vi "Handle Error.vi"(8 "error in (no error)":errorcluster, 11 "IMediator In":refnum<class "IMediator.lvclass">) -> (0 "error out":errorcluster, 2 "stop actor?":bool=TRUE, 3 "IMediator Out":refnum<class "IMediator.lvclass">)   [LabVIEW 2017, in "IMediator.lvlib" / "IMediator.lvclass"]
doc: "(<B>Filename</B>: Actor Framework.lvlib:Actor.lvclass:Handle Error.vi)\n\nDefines how the actor handles an error that occurred while processing a message. By default, this method does nothing except stop the actor."
uses:
  IMediator.lvclass
  gpm_packages/@cs/event-logger/Source/Composed Log/Log Sink/Log Level.ctl
  gpm_packages/@cs/event-logger/Source/Composed Log/Log Sink/Log Sink.lvclass
  gpm_packages/@cs/event-logger/Source/Composed Log/Composed Log.lvlib
  <vilib>/ActorFramework/Actor/Actor.lvclass
  C:/Program Files (x86)/National Instruments/LabVIEW 2017/vi.lib/ActorFramework/Actor/Actor.lvclass
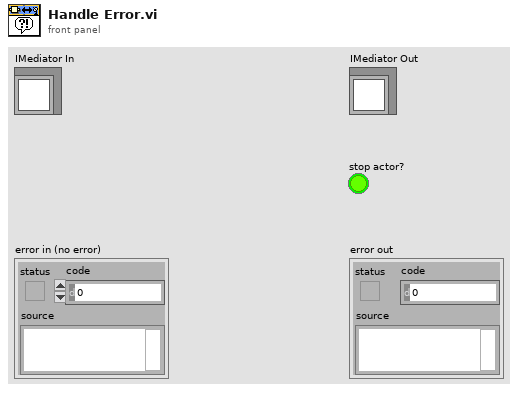
[diagram p1: front panel]
types:
  T1 = typedef "Composed Log.lvlib/Log Sink.lvclass/Log Level.ctl" = enum16{"Debug", "Info", "Warning", "Error", "Critical"}
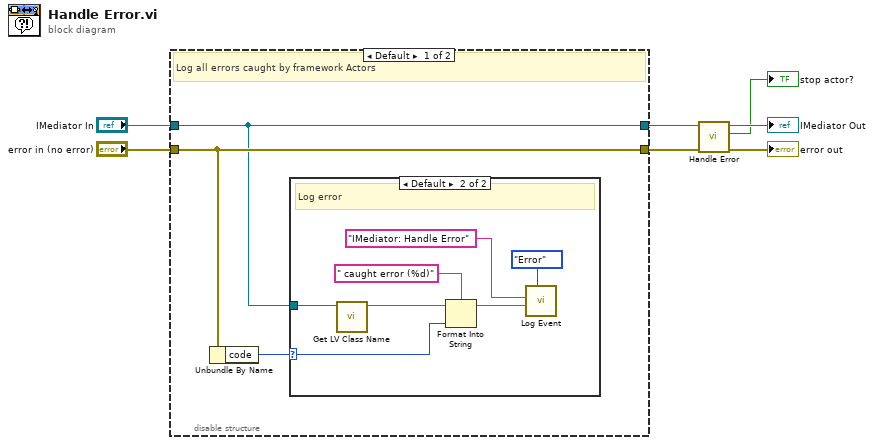
[diagram p0: block diagram]
diagram:
  n1 = disable-structure shown="Default" {
    disable-tunnel: "IMediator In" -> [w8 w19]
    disable-tunnel: [w8 w19] -> w2
    disable-tunnel: "error in (no error)" -> [w10 w18]
    disable-tunnel: [w10 w18] -> w1
    frame condition #0 (active) {
      # "Log all errors caught by framework Actors"
      n2 = Unbundle By Name(w10) -> ("code"=w9:i32)
      n3 = case shown="Default" w9 {
        selector: w9 -> [_ w14]
        tunnel: w8 -> [_ w13]
        frame 43 {
          # "Normal shutdown -- Do not log"
        }
        frame Default {
          # "Log error"
          n4 = call <vilib>:"Get LV Class Name.vi"("object"=w13) -> ("class name"=w16:string)  [unwired: 9 in, 1 out]
          n5 = Format Into String(format string=" caught error (%d)", initial string=w16, w14) -> (resulting string=w11:string)  [unwired: 1 in, 1 out]
          n6 = call "Log Event.vi"("Event Level"=Log_Level."Error", "Data To Log"=w11, "SourceID"="IMediator: Handle Error") -> ()  [unwired: 7 in, 2 out]
        }
      }
    }
    frame condition #1 {
      # "Remove all logging from this method at compile time"
    }
  }
  n7 = call-parent "Handle Error.vi"("error in (no error)"=w1, "Actor in"=w2) -> ("error out"=→"error out":errorcluster, "stop actor?"=→"stop actor?":bool, "Actor out"=→"IMediator Out":refnum<class "IMediator.lvclass">)  [unwired: 7 in]
